vi "reemplazaPuntoDecimal.vi"(1 "Tabla Referencia Acústica Generador Externo in":string[][](array[string])) -> (0 "Tabla Referencia Acústica Generador Externo out":string[][](array[string]))   [LabVIEW 2019, in "Base de Datos.lvclass"]
doc: "cambia el punto decimal hecho con \"coma\" por \"punto\". Esto porque SQLite maneja el punto como punto decimal, y no la coma. La coma la usa para separar distintos comandos."
uses:
  Base de Datos.lvclass
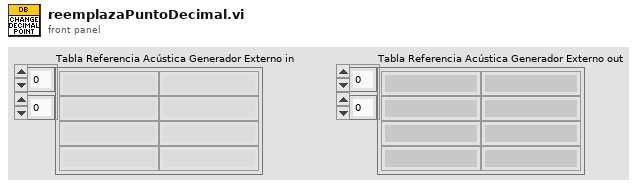
[diagram p1: front panel]
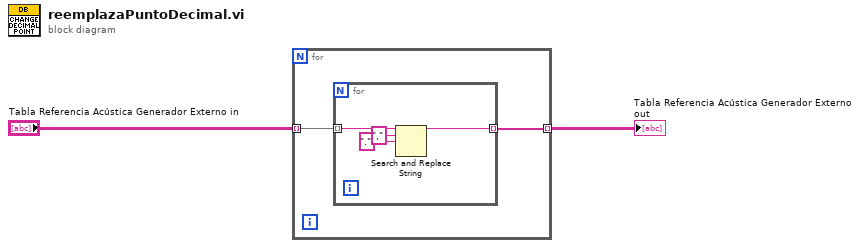
[diagram p0: block diagram]
diagram:
  n1 = for {
    tunnel: "Tabla Referencia Acústica Generador Externo in" -> [w4] mode=indexing
    tunnel: [w3] -> w2 mode=indexing
    n2 = for {
      tunnel: w4 -> [w8] mode=indexing
      tunnel: [w5] -> w3 mode=indexing
      n3 = Search and Replace String(input string=w8, search string=",", replace string="." ("replace string (\"\")")) -> (result string=w5:string)  [unwired: 5 in, 3 out]
    }
  }
  "Tabla Referencia Acústica Generador Externo out" <- w2
